vi "Example Threshold.vi"() -> ()   [LabVIEW 2010]
uses:
  C:/tf/play/labview/Tinkerforge.dll
panel:
  out "last c":i32
  out "last b":i32
  out "last g":i32
  in  "stop":bool
  out "callback counter":i32
  out "last r":i32
  in  "uid":string="abc"
  in  "port":i32=4223
  in  "host":string="localhost"
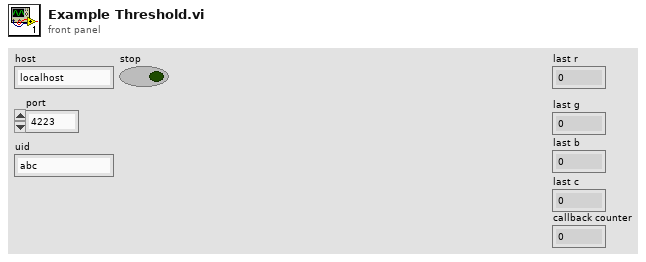
[diagram p1: front panel]
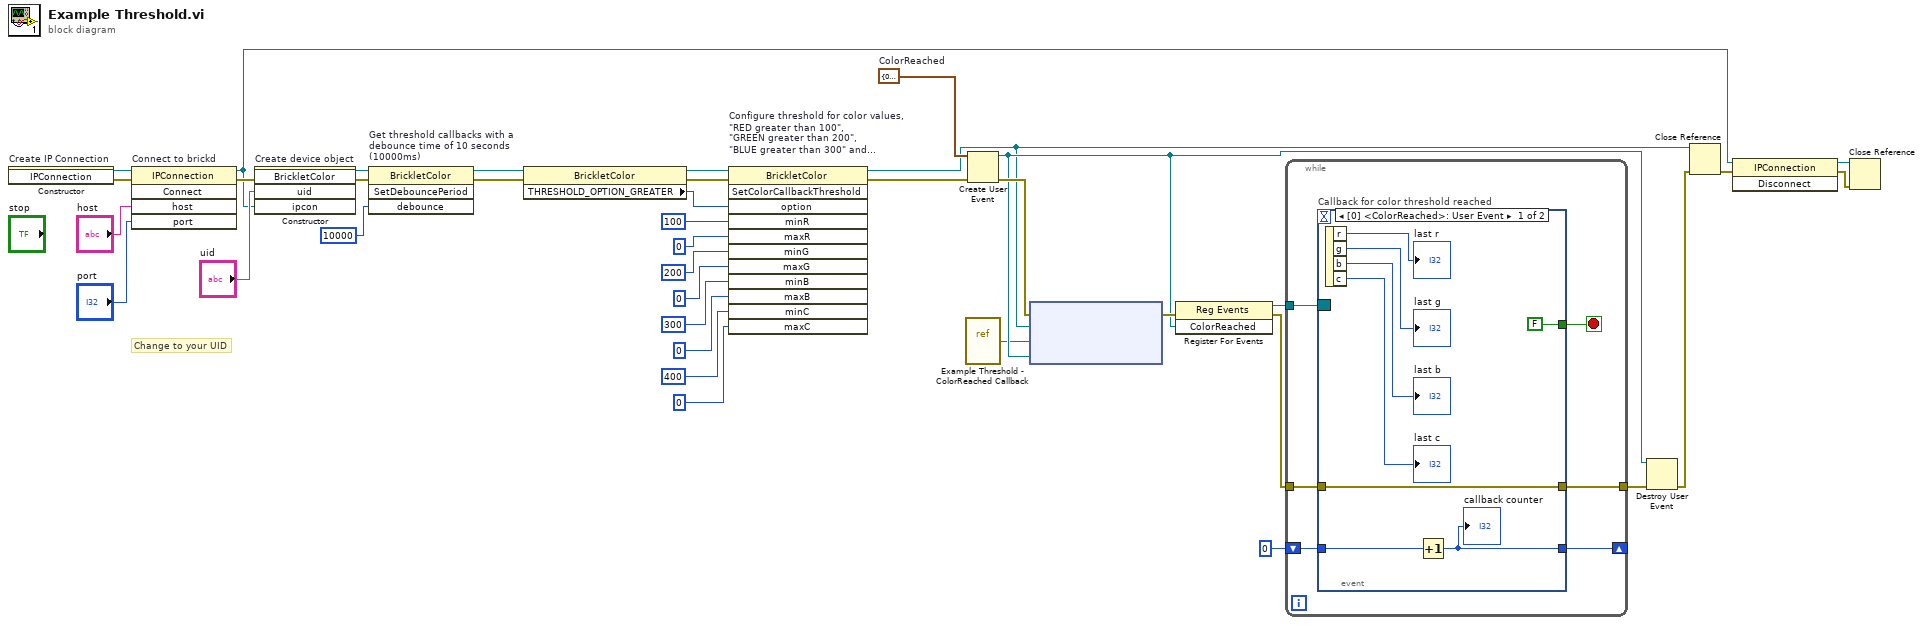
[diagram p0: block diagram]
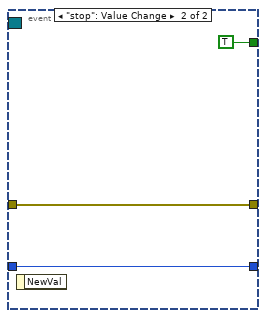
[diagram p2: hidden frame]
diagram:
  w22 = cluster{"r":i32, "g":i32, "b":i32, "c":i32} {"r"=0, "g"=0, "b"=0, "c"=0}  # ColorReached
  # "Change to your UID"
  n1 = constructor on="Create IP Connection" class="IPConnection"() -> (reference out=w38:refnum<k24>, error out=w10:errorcluster)  [unwired: 3 in, 1 out]
  n2 = invoke on="Connect to brickd" class="IPConnection" method="Connect"(reference=w38, error in=w10, "host"="host", "port"="port") -> (reference out=w31:refnum<k24>, error out=w34:errorcluster)  [unwired: 1 in, 3 out]
  n3 = constructor on="Create device object" class="BrickletColor"(error in=w34, "uid"="uid", "ipcon"=w31) -> (reference out=w20:refnum<k24>, error out=w21:errorcluster)  [unwired: 2 in, 3 out]
  n4 = invoke on="Get threshold callbacks with a\ndebounce time of 10 seconds\n(10000ms)" class="BrickletColor" method="SetDebouncePeriod"(reference=w20, error in=w21, "debounce"=i64 10000 ("period")) -> (reference out=w14:refnum<k24>, error out=w16:errorcluster)  [unwired: 1 in, 2 out]
  n5 = property class="BrickletColor"(reference=w14, error in=w16) -> (reference out=w13:refnum<k24>, error out=w15:errorcluster, "THRESHOLD_OPTION_GREATER"=w12:u16)
  n6 = invoke on="Configure threshold for color values,\n\"RED greater than 100\",\n\"GREEN greater than 200\",\n\"BLUE greater than 300\" and\n\"CLEAR greater than 400\"" class="BrickletColor" method="SetColorCallbackThreshold"(reference=w13, error in=w15, "option"=w12, "minR"=100, "maxR"=0, "minG"=200 ("maxR"), "maxG"=0, "minB"=300, "maxB"=0, "minC"=400, "maxC"=0) -> (reference out=w18:refnum<k24>, error out=w17:errorcluster)  [unwired: 1 in, 10 out]
  n7 = vi-ref "Example Threshold - ColorReached Callback.vi"() -> ("vi reference"=w1:refnum<vi>)
  n8 = Create User Event(user event datatype=w22, error in=w17) -> (user event=w24:refnum<user-event>, error out=w29:errorcluster)
  n9 = node ("Register Event Callback")(w29, w18, w1, w24) -> (w28:errorcluster)  [unwired: 1 in, 1 out]
  n10 = register-events(error in=w28, w24) -> (reference out=w27:refnum<event-registration>, error out=w25:errorcluster)  [unwired: 1 in]
  n11 = while {
    tunnel: w27 -> [w44]
    tunnel: [w43] -> w26
    tunnel: w25 -> [w42]
    shift-right: [w40] -> _
    shift-left: 0 -> [w41]
    stop <- w39 stop-if-true
    n12 = event "Callback for color threshold reached" shown="[0] <ColorReached>: User Event" {
      selector: w44 -> [_ _]
      dyn-events: _ -> [_ _]
      timeout: _ -> [_ _]
      tunnel: [w52 w54] -> w43
      tunnel: w42 -> [w52 w54]
      tunnel: w41 -> [w51 w53]
      tunnel: [w50 w53] -> w40
      tunnel: [FALSE TRUE] -> w39
      event User Event {
        n13 = event-data() -> ("r"=→"last r":i32, "g"=→"last g":i32, "b"=→"last b":i32, "c"=→"last c":i32)  [unwired: 1 in]
        n14 = Increment(x=w51) -> (x+1=w50:i32)
        "callback counter" <- w50
      }
      event "stop": Value Change {
        n15 = event-data() -> ()  [unwired: 1 in, 1 out]
      }
    }
  }
  n16 = Destroy User Event(user event=w24, error in=w26) -> (error out=w23:errorcluster)
  n17 = Close Reference(reference=w18, error in (no error)=w23) -> (error out=w33:errorcluster)
  n18 = invoke class="IPConnection" method="Disconnect"(reference=w31, error in=w33) -> (reference out=w30:refnum<k24>, error out=w32:errorcluster)  [unwired: 1 in, 1 out]
  n19 = Close Reference(reference=w30, error in (no error)=w32) -> ()  [unwired: 1 out]
